vi "Read_raw_meas_setup.vi"(8 "Setup file string":string) -> (0 "No of Blocks":i32=1, 1 "Sampling freq (Hz)":dbl=100.0, 2 "No of samples":i32=500 min=0 step=1, 3 "Analysis Info cluster 2":T1[](array[typedef])=[{"Colour"=0, "Inst type"=enum."Pitot-static tube", "Inst name"="Manometer voltage", "Symbol"="U", "Code name"="", "Extra Info"="U", "Inst Array"=enum."PWA", "Extra Titles"=[], "Extra Values"=[], "U"=0.0, "u^2"=0.0, "u^3"=0.0, "u^4"=0.0, "Skew_u"=0.0, "Kurt_u"=0.0, "Sd Error in Mean"=0.0, "% u'/U"=0.0, "X"=0.0, "Y"=0.0, "Z"=0.0, "Timescale integral to 25%"=0.0, "Sd Error in Variance"=0.0, "Calib File"=path "", "Calib Constants"=[], "Output Position"=FALSE, "Full Stats"=FALSE, "Av Sampling Rate"=0.0, "Av No of Samples"=0.0, "Total Meas Time (s)"=0.0, "ADAM Ch Name"=""}, {"Colour"=0, "Inst type"=enum."Pitot-static tube", "Inst name"="Manometer voltage", "Symbol"="U", "Code name"="", "Extra Info"="U", "Inst Array"=enum."PWA", "Extra Titles"=[], "Extra Values"=[], "U"=0.0, "u^2"=0.0, "u^3"=0.0, "u^4"=0.0, "Skew_u"=0.0, "Kurt_u"=0.0, "Sd Error in Mean"=0.0, "% u'/U"=0.0, "X"=0.0, "Y"=0.0, "Z"=0.0, "Timescale integral to 25%"=0.0, "Sd Error in Variance"=0.0, "Calib File"=path "", "Calib Constants"=[], "Output Position"=FALSE, "Full Stats"=FALSE, "Av Sampling Rate"=0.0, "Av No of Samples"=0.0, "Total Meas Time (s)"=0.0, "ADAM Ch Name"=""}, {"Colour"=0, "Inst type"=enum."Pitot-static tube", "Inst name"="Manometer voltage", "Symbol"="U", "Code name"="", "Extra Info"="U", "Inst Array"=enum."PWA", "Extra Titles"=[], "Extra Values"=[], "U"=0.0, "u^2"=0.0, "u^3"=0.0, "u^4"=0.0, "Skew_u"=0.0, "Kurt_u"=0.0, "Sd Error in Mean"=0.0, "% u'/U"=0.0, "X"=0.0, "Y"=0.0, "Z"=0.0, "Timescale integral to 25%"=0.0, "Sd Error in Variance"=0.0, "Calib File"=path "", "Calib Constants"=[], "Output Position"=FALSE, "Full Stats"=FALSE, "Av Sampling Rate"=0.0, "Av No of Samples"=0.0, "Total Meas Time (s)"=0.0, "ADAM Ch Name"=""}, {"Colour"=0, "Inst type"=enum."Pitot-static tube", "Inst name"="Manometer voltage", "Symbol"="U", "Code name"="", "Extra Info"="U", "Inst Array"=enum."PWA", "Extra Titles"=[], "Extra Values"=[], "U"=0.0, "u^2"=0.0, "u^3"=0.0, "u^4"=0.0, "Skew_u"=0.0, "Kurt_u"=0.0, "Sd Error in Mean"=0.0, "% u'/U"=0.0, "X"=0.0, "Y"=0.0, "Z"=0.0, "Timescale integral to 25%"=0.0, "Sd Error in Variance"=0.0, "Calib File"=path "", "Calib Constants"=[], "Output Position"=FALSE, "Full Stats"=FALSE, "Av Sampling Rate"=0.0, "Av No of Samples"=0.0, "Total Meas Time (s)"=0.0, "ADAM Ch Name"=""}] {"Sd Error in Variance" format="%.2f"; "Skew_u" format="%.2f"; "% u'/U" format="%.2f"; "Sd Error in Mean" format="%.2f"; "Kurt_u" format="%.2f"; "u^4" format="%.2f"; "u^3" format="%.2f"; "U" format="%.2f"; "u^2" format="%.2f"})   [LabVIEW 2015]
uses:
  Controls/Analysis_info_cluster.ctl
  Controls/Inst_type.ctl
  Controls/Instrument_Array.ctl
  Globals/Meas_global.vi
  Globals/LDA_meas_global_1.vi
  Globals/LDA_meas_global_2.vi
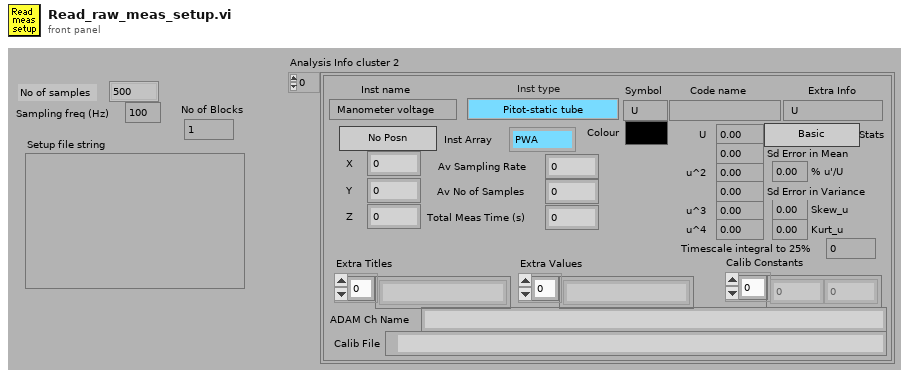
[diagram p1: front panel]
types:
  T1 = typedef "Analysis_info_cluster.ctl" = cluster{"Colour":u32, "Inst type":T2, "Inst name":string, "Symbol":string, "Code name":string, "Extra Info":string, "Inst Array":T3, "Extra Titles":string[], "Extra Values":string[], "U":dbl, "u^2":dbl, "u^3":dbl, "u^4":dbl, "Skew_u":dbl, "Kurt_u":dbl, "Sd Error in Mean":dbl, "% u'/U":dbl, "X":dbl, "Y":dbl, "Z":dbl, "Timescale integral to 25%":dbl, "Sd Error in Variance":dbl, "Calib File":path, "Calib Constants":dbl[], "Output Position":bool, "Full Stats":bool, "Av Sampling Rate":dbl, "Av No of Samples":dbl, "Total Meas Time (s)":dbl, "ADAM Ch Name":string}
  T2 = typedef "Inst_type.ctl" = enum16{"Propeller anemometer", "Raw voltage", "Pressure Transducer", "Pitot-static tube", "Preston tube", "Hot wire", "Cross wire 1", "Cross wire 2", "Generic Linear", "Generic Polynomial", "Generic BackPoly", "Fast FID", "Thermocouple", "Cold wire", "Pulsed Wire", "LDA Vel", "LDA Tran time", "LDA Arr time", "Microphone"}
  T3 = typedef "Instrument_Array.ctl" = enum16{"PWA", "LDA", "Analogue"}
  T4 = typedef "Post_Process.ctl" = enum16{"Take New Data", "Post Process Raw Data File"}
  T5 = enum16{"From String to Cluster", "From Cluster to String"}
  T6 = typedef "BSA_Type.ctl" = enum16{"57N11", "BSA F60"}
  T7 = typedef "LDA_Setup.ctl" = cluster{"dimensions":enum16{"1D", "2D"}, "Analogue Freq Multiplier":dbl}
  T8 = typedef "BSA_info_Cluster.ctl" = cluster{"GPIB Address":string, "No of Check Bytes":i32, "Extra Info":string, "COLOUR":u32, "Wavelength (nm)":dbl}
  T9 = typedef "Graph_Type.ctl" = enum16{"Show no graph", "Voltage trace", "Velocity trace", "Vel histogram", "Spectrum", "f.E(f) v Log f", "Auto-Corr"}
  T10 = cluster{"Plot 1":u16, "Plot 2":u16, "Save graph":u16, "Plot Type":T9}
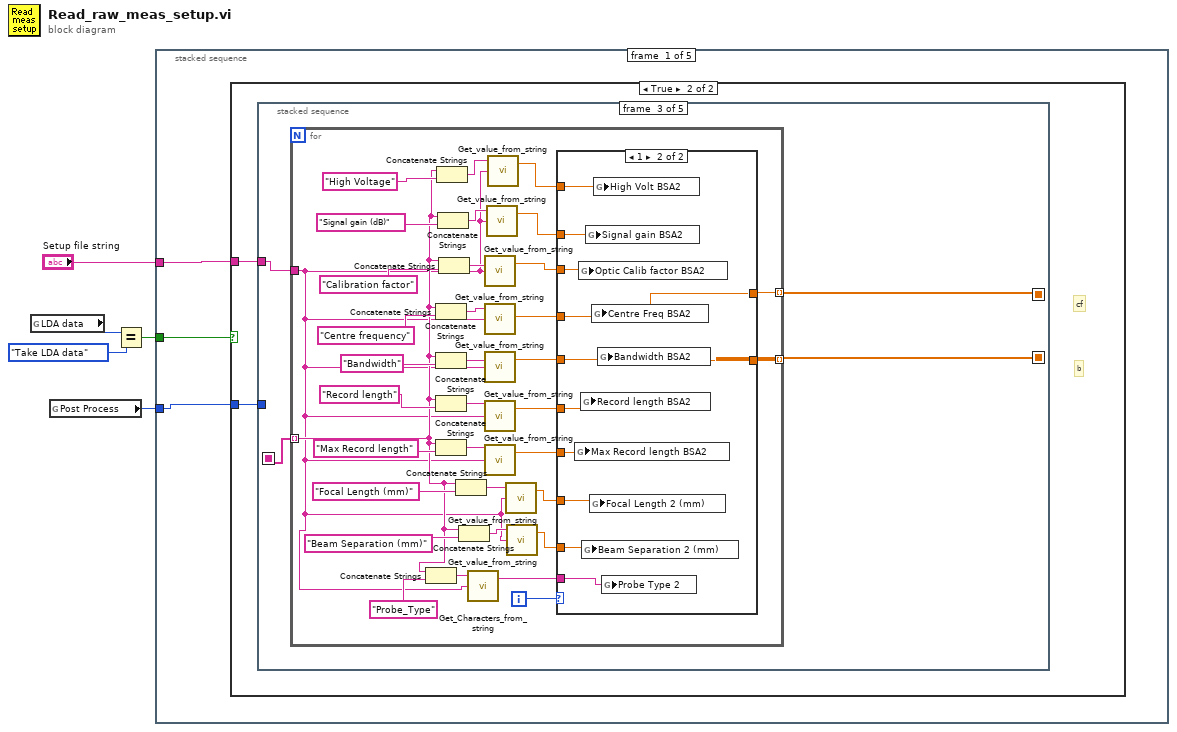
[diagram p0: block diagram]
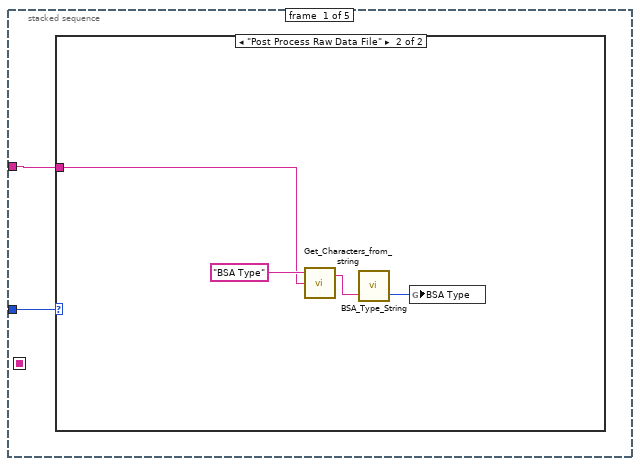
[diagram p3: hidden frame]
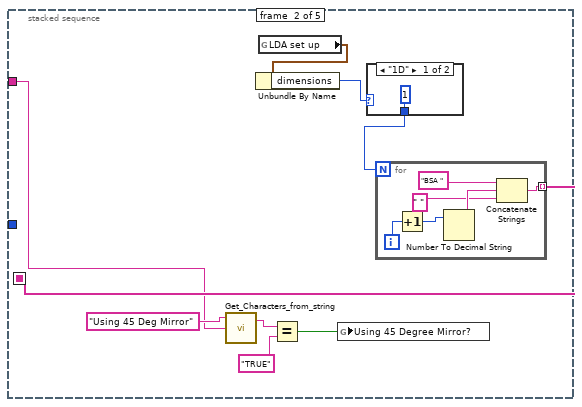
[diagram p5: hidden frame]
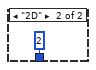
[diagram p6: hidden frame]
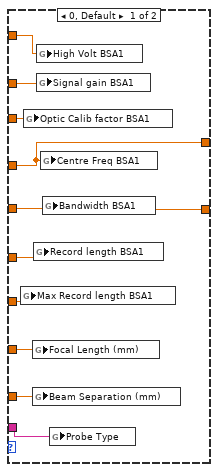
[diagram p7: hidden frame]
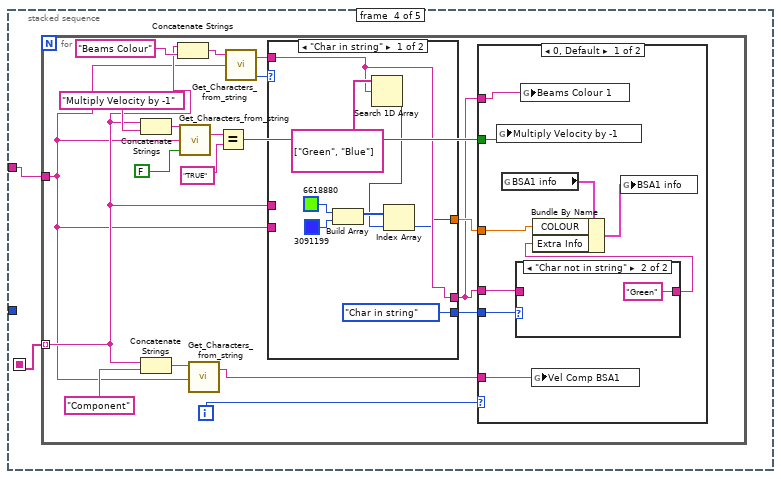
[diagram p8: hidden frame]
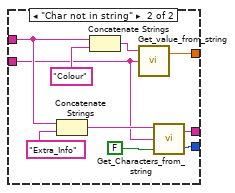
[diagram p9: hidden frame]
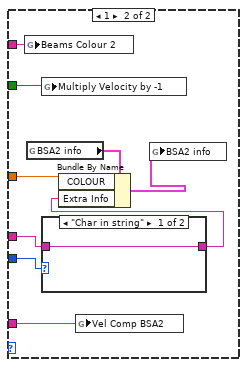
[diagram p11: hidden frame]
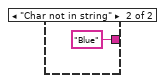
[diagram p12: hidden frame]
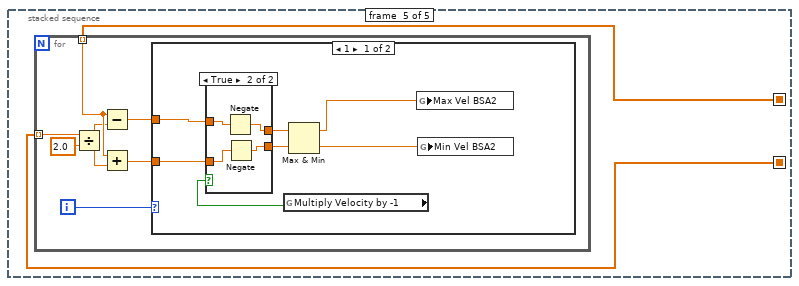
[diagram p13: hidden frame]
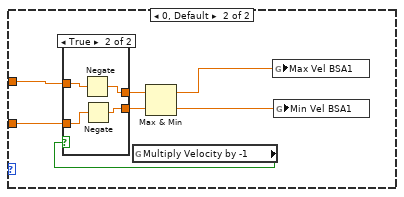
[diagram p15: hidden frame]
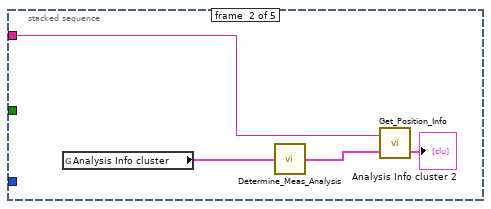
[diagram p17: hidden frame]
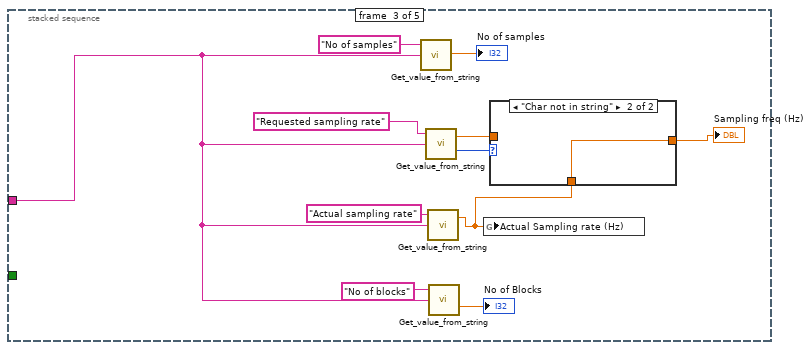
[diagram p18: hidden frame]
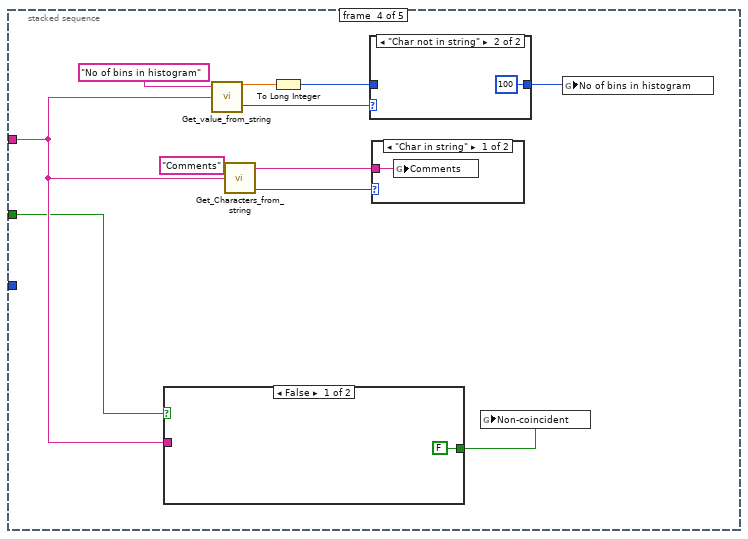
[diagram p20: hidden frame]
diagram:
  n1 = global read "Meas_global.vi" "LDA data"() -> (w3:enum16{"No LDA data", "Take LDA data"})
  n2 = global read "Meas_global.vi" "Post Process"() -> (w5:T4)
  n3 = Equal?(x=w3, y=enum16{"No LDA data", "Take LDA data"}."Take LDA data" ("LDA data")) -> (x = y?=w2:bool)
  n4 = stacked-sequence {
    tunnel: w5 -> [w6 _ _ _ _]
    tunnel: w2 -> [w8 _ _ w206 _]
    tunnel: "Setup file string" -> [w7 w192 w198 w207 w226]
    frame #0 {
      n5 = case shown="True" w8 {
        tunnel: w7 -> [_ w10]
        tunnel: w6 -> [_ w9]
        frame False {
        }
        frame True {
          # "b"
          # "cf"
          n6 = stacked-sequence {
            seq-local: [_ w24 _ _ _] -> [_ _ w36 w93 _]
            seq-local: [_ _ w34 _ _] -> [_ _ _ _ w154]
            seq-local: [_ _ w35 _ _] -> [_ _ _ _ w155]
            tunnel: w10 -> [w11 w18 w37 w94 _]
            tunnel: w9 -> [w12 _ _ _ _]
            frame #0 {
              n7 = case shown="\"Post Process Raw Data File\"" w12 {
                tunnel: w11 -> [_ w13]
                frame "Take New Data" {
                }
                frame "Post Process Raw Data File" {
                  n8 = call "Get_Characters_from_string.vi"("Input string"=w13, "Variable name"="BSA Type" ("Label for characters")) -> ("Value"=w15:string)  [unwired: 1 in, 1 out]
                  n9 = call "BSA_Type_String.vi"("BSA String in"=w15) -> ("BSA Type Out"=w14:T6)  [unwired: 1 in, 1 out]
                  n10 = global write "LDA_meas_global_1.vi" "BSA Type"(w14) -> ()
                }
              }
            }
            frame #1 {
              n11 = call "Get_Characters_from_string.vi"("Input string"=w18, "Variable name"="Using 45 Deg Mirror") -> ("Value"=w21:string)  [unwired: 1 in, 1 out]
              n12 = global read "Meas_global.vi" "LDA set up"() -> (w23:T7)
              n13 = Unbundle By Name(w23) -> ("dimensions"=w22:enum16{"1D", "2D"})
              n14 = Equal?(x=w21, y="TRUE") -> (x = y?=w17:bool)
              n15 = global write "LDA_meas_global_1.vi" "Using 45 Degree Mirror?"(w17) -> ()
              n16 = case shown="\"1D\"" w22 {
                tunnel: [1 2] -> w25
                frame "1D" {
                }
                frame "2D" {
                }
              }
              n17 = for {
                N: w25 -> [_]
                tunnel: [w27] -> w24 mode=indexing
                i -> [w29]
                n18 = Increment(x=w29) -> (x+1=w28:i32)
                n19 = Number To Decimal String(number=w28) -> (decimal integer string=w31:string)  [unwired: 1 out]
                n20 = Concatenate Strings("BSA ", w31, " ") -> (w27:string)
              }
            }
            frame #2 {
              n21 = for {
                tunnel: w37 -> [w39]
                tunnel: w36 -> [w42] mode=indexing
                tunnel: [w60] -> w35 mode=indexing
                tunnel: [w59] -> w34 mode=indexing
                i -> [w64]
                n22 = Concatenate Strings(w42, "Probe_Type" ("Label for characters")) -> (w40:string)
                n23 = Concatenate Strings(w42, "Centre frequency") -> (w67:string)
                n24 = Concatenate Strings(w42, "Bandwidth") -> (w66:string)
                n25 = Concatenate Strings(w42, "Record length") -> (w65:string)
                n26 = Concatenate Strings(w42, "Max Record length") -> (w50:string)
                n27 = Concatenate Strings(w42, "High Voltage") -> (w54:string)
                n28 = Concatenate Strings(w42, "Signal gain (dB)") -> (w55:string)
                n29 = Concatenate Strings(w42, "Calibration factor") -> (w68:string)
                n30 = Concatenate Strings(w42, "Focal Length (mm)" ("Label for characters")) -> (w47:string)
                n31 = Concatenate Strings(w42, "Beam Separation (mm)" ("Label for characters")) -> (w48:string)
                n32 = call "Get_Characters_from_string.vi"("Input string"=w39, "Variable name"=w40) -> ("Value"=w38:string)  [unwired: 1 in, 1 out]
                n33 = call "Get_value_from_string.vi"("Input string"=w39, "Variable name"=w68) -> ("Value"=w58:dbl)  [unwired: 1 in, 1 out]
                n34 = call "Get_value_from_string.vi"("Input string"=w39, "Variable name"=w67) -> ("Value"=w63:dbl)  [unwired: 1 in, 1 out]
                n35 = call "Get_value_from_string.vi"("Input string"=w39, "Variable name"=w66) -> ("Value"=w62:dbl)  [unwired: 1 in, 1 out]
                n36 = call "Get_value_from_string.vi"("Input string"=w39, "Variable name"=w65) -> ("Value"=w61:dbl)  [unwired: 1 in, 1 out]
                n37 = call "Get_value_from_string.vi"("Input string"=w39, "Variable name"=w50) -> ("Value"=w51:dbl)  [unwired: 1 in, 1 out]
                n38 = call "Get_value_from_string.vi"("Input string"=w39, "Variable name"=w55) -> ("Value"=w53:dbl)  [unwired: 1 in, 1 out]
                n39 = call "Get_value_from_string.vi"("Input string"=w39, "Variable name"=w54) -> ("Value"=w52:dbl)  [unwired: 1 in, 1 out]
                n40 = call "Get_value_from_string.vi"("Input string"=w39, "Variable name"=w47) -> ("Value"=w44:dbl)  [unwired: 1 in, 1 out]
                n41 = call "Get_value_from_string.vi"("Input string"=w39, "Variable name"=w48) -> ("Value"=w43:dbl)  [unwired: 1 in, 1 out]
                n42 = case shown="1" w64 {
                  tunnel: w63 -> [w79 w90]
                  tunnel: w62 -> [w80 w89]
                  tunnel: w61 -> [w81 w92]
                  tunnel: w58 -> [w82 w91]
                  tunnel: [w80 w89] -> w60
                  tunnel: [w79 w90] -> w59
                  tunnel: w53 -> [w78 w87]
                  tunnel: w52 -> [w77 w88]
                  tunnel: w51 -> [w76 w86]
                  tunnel: w44 -> [w75 w85]
                  tunnel: w43 -> [w74 w84]
                  tunnel: w38 -> [w73 w83]
                  frame 0, Default {
                    n43 = global write "LDA_meas_global_1.vi" "Max Record length BSA1"(w76) -> ()
                    n44 = global write "LDA_meas_global_1.vi" "Optic Calib factor BSA1"(w82) -> ()
                    n45 = global write "LDA_meas_global_1.vi" "Focal Length (mm)"(w75) -> ()
                    n46 = global write "LDA_meas_global_1.vi" "Beam Separation (mm)"(w74) -> ()
                    n47 = global write "LDA_meas_global_1.vi" "Record length BSA1"(w81) -> ()
                    n48 = global write "LDA_meas_global_1.vi" "High Volt BSA1"(w77) -> ()
                    n49 = global write "LDA_meas_global_1.vi" "Signal gain BSA1"(w78) -> ()
                    n50 = global write "LDA_meas_global_1.vi" "Centre Freq BSA1"(w79) -> ()
                    n51 = global write "LDA_meas_global_1.vi" "Bandwidth BSA1"(w80) -> ()
                    n52 = global write "LDA_meas_global_1.vi" "Probe Type"(w73) -> ()
                  }
                  frame 1 {
                    n53 = global write "LDA_meas_global_2.vi" "Max Record length BSA2"(w86) -> ()
                    n54 = global write "LDA_meas_global_2.vi" "Optic Calib factor BSA2"(w91) -> ()
                    n55 = global write "LDA_meas_global_2.vi" "Record length BSA2"(w92) -> ()
                    n56 = global write "LDA_meas_global_2.vi" "Beam Separation 2 (mm)"(w84) -> ()
                    n57 = global write "LDA_meas_global_2.vi" "Signal gain BSA2"(w87) -> ()
                    n58 = global write "LDA_meas_global_2.vi" "Focal Length 2 (mm)"(w85) -> ()
                    n59 = global write "LDA_meas_global_2.vi" "Centre Freq BSA2"(w90) -> ()
                    n60 = global write "LDA_meas_global_2.vi" "High Volt BSA2"(w88) -> ()
                    n61 = global write "LDA_meas_global_2.vi" "Bandwidth BSA2"(w89) -> ()
                    n62 = global write "LDA_meas_global_2.vi" "Probe Type 2"(w83) -> ()
                  }
                }
              }
            }
            frame #3 {
              n63 = for {
                tunnel: w94 -> [w98]
                tunnel: w93 -> [w99] mode=indexing
                i -> [w112]
                n64 = Concatenate Strings(w99, "Multiply Velocity by -1") -> (w109:string)
                n65 = Concatenate Strings(w99, "Component") -> (w113:string)
                n66 = Concatenate Strings(w99, "Beams Colour") -> (w102:string)
                n67 = call "Get_Characters_from_string.vi"("Show Dialog?"=FALSE, "Input string"=w98, "Variable name"=w109) -> ("Value"=w107:string)  [unwired: 1 out]
                n68 = call "Get_Characters_from_string.vi"("Input string"=w98, "Variable name"=w113) -> ("Value"=w110:string)  [unwired: 1 in, 1 out]
                n69 = Equal?(x=w107, y="TRUE") -> (x = y?=w105:bool)
                n70 = call "Get_Characters_from_string.vi"("Input string"=w98, "Variable name"=w102) -> ("Status"=w97:enum16{"Char in string", "Char not in string"}, "Value"=w96:string)  [unwired: 1 in]
                n71 = case shown="\"Char in string\"" w97 {
                  tunnel: [enum16{"Char in string", "Char not in string"}."Char in string" ("Status") w128] -> w104
                  tunnel: [w114 w127] -> w100
                  tunnel: [w116 w124] -> w95
                  tunnel: w99 -> [_ w123]
                  tunnel: w98 -> [_ w122]
                  tunnel: w96 -> [w116 _]
                  frame "Char in string" {
                    n72 = Build Array(u32 6618880, u32 3091199) -> (w118:u32[])
                    n73 = Search 1D Array(1D array=string[] ["Green", "Blue"], element=w116) -> (index of element=w117:i32)  [unwired: 1 in]
                    n74 = Index Array(array=w118, index=w117) -> (element=w114:u32)
                  }
                  frame "Char not in string" {
                    n75 = Concatenate Strings(w123, "Extra_Info" ("string")) -> (w131:string)
                    n76 = Concatenate Strings(w123, "Colour") -> (w125:string)
                    n77 = call "Get_value_from_string.vi"("Input string"=w122, "Variable name"=w125) -> ("Value"=w127:dbl)  [unwired: 1 in, 1 out]
                    n78 = call "Get_Characters_from_string.vi"("Show Dialog?"=FALSE, "Input string"=w122, "Variable name"=w131) -> ("Status"=w128:enum16{"Char in string", "Char not in string"}, "Value"=w124:string)
                  }
                }
                n79 = case shown="0, Default" w112 {
                  tunnel: w100 -> [w139 w150]
                  tunnel: w110 -> [w138 w149]
                  tunnel: w105 -> [w137 w148]
                  tunnel: w104 -> [w136 w145]
                  tunnel: w95 -> [w135 w146]
                  tunnel: w95 -> [w132 w143]
                  frame 0, Default {
                    n80 = global write "LDA_meas_global_1.vi" "Multiply Velocity by -1"(w137) -> ()
                    n81 = global read "LDA_meas_global_1.vi" "BSA1 info"() -> (w140:T8)
                    n82 = case shown="\"Char not in string\"" w136 {
                      tunnel: w135 -> [w141 _]
                      tunnel: [w141 "Green" ("Value")] -> w133
                      frame "Char in string" {
                      }
                      frame "Char not in string" {
                      }
                    }
                    n83 = global write "LDA_meas_global_1.vi" "Beams Colour 1"(w132) -> ()
                    n84 = global write "LDA_meas_global_1.vi" "Vel Comp BSA1"(w138) -> ()
                    n85 = Bundle By Name(cluster=w140, "COLOUR"=w139, "Extra Info"=w133) -> (w134:T8)
                    n86 = global write "LDA_meas_global_1.vi" "BSA1 info"(w134) -> ()
                  }
                  frame 1 {
                    n87 = global write "LDA_meas_global_2.vi" "Beams Colour 2"(w143) -> ()
                    n88 = global read "LDA_meas_global_2.vi" "BSA2 info"() -> (w151:T8)
                    n89 = global write "LDA_meas_global_2.vi" "Multiply Velocity by -1"(w148) -> ()
                    n90 = case shown="\"Char in string\"" w145 {
                      tunnel: w146 -> [w152 _]
                      tunnel: [w152 "Blue" ("Value")] -> w144
                      frame "Char in string" {
                      }
                      frame "Char not in string" {
                      }
                    }
                    n91 = Bundle By Name(cluster=w151, "COLOUR"=w150, "Extra Info"=w144) -> (w147:T8)
                    n92 = global write "LDA_meas_global_2.vi" "Vel Comp BSA2"(w149) -> ()
                    n93 = global write "LDA_meas_global_2.vi" "BSA2 info"(w147) -> ()
                  }
                }
              }
            }
            frame #4 {
              n94 = for {
                tunnel: w155 -> [w161] mode=indexing
                tunnel: w154 -> [w160] mode=indexing
                i -> [w156]
                n95 = Divide(x=w161, y=2.0) -> (x/y=w159:dbl)
                n96 = Subtract(x=w160, y=w159) -> (x-y=w157:dbl)
                n97 = Add(x=w160, y=w159) -> (x+y=w158:dbl)
                n98 = case shown="1" w156 {
                  tunnel: w158 -> [w169 w182]
                  tunnel: w157 -> [w168 w181]
                  frame 1 {
                    n99 = global read "LDA_meas_global_2.vi" "Multiply Velocity by -1"() -> (w165:bool)
                    n100 = case shown="True" w165 {
                      tunnel: w169 -> [w170 w175]
                      tunnel: w168 -> [w171 w174]
                      tunnel: [w171 w173] -> w167
                      tunnel: [w170 w172] -> w166
                      frame False {
                      }
                      frame True {
                        n101 = Negate(x=w174) -> (-x=w173:dbl)
                        n102 = Negate(x=w175) -> (-x=w172:dbl)
                      }
                    }
                    n103 = Max & Min(x=w167, y=w166) -> (max(x,y)=w163:dbl, min(x,y)=w164:dbl)
                    n104 = global write "LDA_meas_global_2.vi" "Max Vel BSA2"(w163) -> ()
                    n105 = global write "LDA_meas_global_2.vi" "Min Vel BSA2"(w164) -> ()
                  }
                  frame 0, Default {
                    n106 = global read "LDA_meas_global_1.vi" "Multiply Velocity by -1"() -> (w178:bool)
                    n107 = case shown="True" w178 {
                      tunnel: w182 -> [w183 w188]
                      tunnel: w181 -> [w184 w187]
                      tunnel: [w184 w186] -> w180
                      tunnel: [w183 w185] -> w179
                      frame False {
                      }
                      frame True {
                        n108 = Negate(x=w187) -> (-x=w186:dbl)
                        n109 = Negate(x=w188) -> (-x=w185:dbl)
                      }
                    }
                    n110 = Max & Min(x=w180, y=w179) -> (max(x,y)=w176:dbl, min(x,y)=w177:dbl)
                    n111 = global write "LDA_meas_global_1.vi" "Max Vel BSA1"(w176) -> ()
                    n112 = global write "LDA_meas_global_1.vi" "Min Vel BSA1"(w177) -> ()
                  }
                }
              }
            }
          }
        }
      }
    }
    frame #1 {
      n113 = global read "Meas_global.vi" "Analysis Info cluster"() -> (w190:T1[])
      n114 = call "Determine_Meas_Analysis.vi"("Analysis info Cluster In"=w190) -> ("Analysis info Cluster Out"=w189:T1[])
      n115 = call "Get_Position_Info.vi"("Analysis Info cluster"=w189, "Setup file string"=w192) -> ("Analysis Info cluster 2"=→"Analysis Info cluster 2":T1[])  [unwired: 1 in]
    }
    frame #2 {
      n116 = call "Get_value_from_string.vi"("Input string"=w198, "Variable name"="No of samples") -> ("Value"=→"No of samples":dbl)  [unwired: 1 in, 1 out]
      n117 = call "Get_value_from_string.vi"("Input string"=w198, "Variable name"="Requested sampling rate") -> ("Status"=w196:enum16{"Char in string", "Char not in string"}, "Value"=w194:dbl)  [unwired: 1 in]
      n118 = call "Get_value_from_string.vi"("Input string"=w198, "Variable name"="Actual sampling rate") -> ("Value"=w193:dbl)  [unwired: 1 in, 1 out]
      n119 = call "Get_value_from_string.vi"("Input string"=w198, "Variable name"="No of blocks") -> ("Value"=→"No of Blocks":dbl)  [unwired: 1 in, 1 out]
      n120 = global write "Meas_global.vi" "Actual Sampling rate (Hz)"(w193) -> ()
      n121 = case shown="\"Char not in string\"" w196 {
        tunnel: [w204 w205] -> w195
        tunnel: w194 -> [w204 _]
        tunnel: w193 -> [_ w205]
        frame "Char in string" {
        }
        frame "Char not in string" {
        }
      }
      "Sampling freq (Hz)" <- w195
    }
    frame #3 {
      n122 = case shown="False" w206 {
        tunnel: [FALSE w219] -> w208
        tunnel: w207 -> [_ w218]
        frame False {
        }
        frame True {
          n123 = call "Get_Characters_from_string.vi"("Input string"=w218, "Variable name"="Non-Coincident Mode" ("Pre Setup String")) -> ("Value"=w221:string)  [unwired: 1 in, 1 out]
          n124 = Equal?(x=w221, y="TRUE") -> (x = y?=w219:bool)
        }
      }
      n125 = call "Get_value_from_string.vi"("Input string"=w207, "Variable name"="No of bins in histogram") -> ("Status"=w215:enum16{"Char in string", "Char not in string"}, "Value"=w214:dbl)  [unwired: 1 in]
      n126 = call "Get_Characters_from_string.vi"("Input string"=w207, "Variable name"="Comments") -> ("Status"=w212:enum16{"Char in string", "Char not in string"}, "Value"=w211:string)  [unwired: 1 in]
      n127 = To Long Integer(number=w214) -> (32bit integer=w213:i32)
      n128 = case shown="\"Char not in string\"" w215 {
        tunnel: w213 -> [w224 _]
        tunnel: [w224 100] -> w209
        frame "Char in string" {
        }
        frame "Char not in string" {
        }
      }
      n129 = case shown="\"Char in string\"" w212 {
        tunnel: w211 -> [w223 _]
        frame "Char in string" {
          n130 = global write "Meas_global.vi" "Comments"(w223) -> ()
        }
        frame "Char not in string" {
        }
      }
      n131 = global write "LDA_meas_global_1.vi" "Non-coincident"(w208) -> ()
      n132 = global write "Meas_global.vi" "No of bins in histogram"(w209) -> ()
    }
    frame #4 {
      n133 = call "Save_Load_Graph_Setup.vi"("Setup String in"=w226, "Graph Number"=1, "Mode"=T5."From String to Cluster") -> ("Variables found?"=w232:bool, "Graph Out"=w231:T10)  [unwired: 1 in, 1 out]
      n134 = call "Save_Load_Graph_Setup.vi"("Setup String in"=w226, "Graph Number"=2, "Mode"=T5."From String to Cluster") -> ("Variables found?"=w228:bool, "Graph Out"=w227:T10)  [unwired: 1 in, 1 out]
      n135 = case shown="True" w232 {
        tunnel: w231 -> [_ w236]
        frame False {
        }
        frame True {
          n136 = global write "Meas_global.vi" "First Graph"(w236) -> ()
        }
      }
      n137 = case shown="True" w228 {
        tunnel: w227 -> [_ w235]
        frame False {
        }
        frame True {
          n138 = global write "Meas_global.vi" "Second Graph"(w235) -> ()
        }
      }
    }
  }
